vi "stepper driver -- IMS -- V2.vi"(7 "stepper driver action":T3, 8 "internal stepper driver state IMS":T1={"VISA address"="GPIB0::25::INSTR", "stepper motor state"=enum."stopped", "Motor Address"=0, "speed"=0, "target position"=0.0, "current position"=0.0}, 11 "number":dbl format="%#_13g") -> (0 "internal stepper driver state IMS -- OUT":T1={"VISA address"="GPIB0::25::INSTR", "stepper motor state"=enum."stopped", "Motor Address"=0, "speed"=0, "target position"=0.0, "current position"=0.0}, 1 "stepper motor state OUT":T2, 3 "current position":dbl)   [LabVIEW 2018]
uses:
  stepper motor action.ctl
  stepper motor state.ctl
  internal stepper driver state -- IMS.ctl
  stack action -- control.ctl
  Q - not nan -- integer.vi
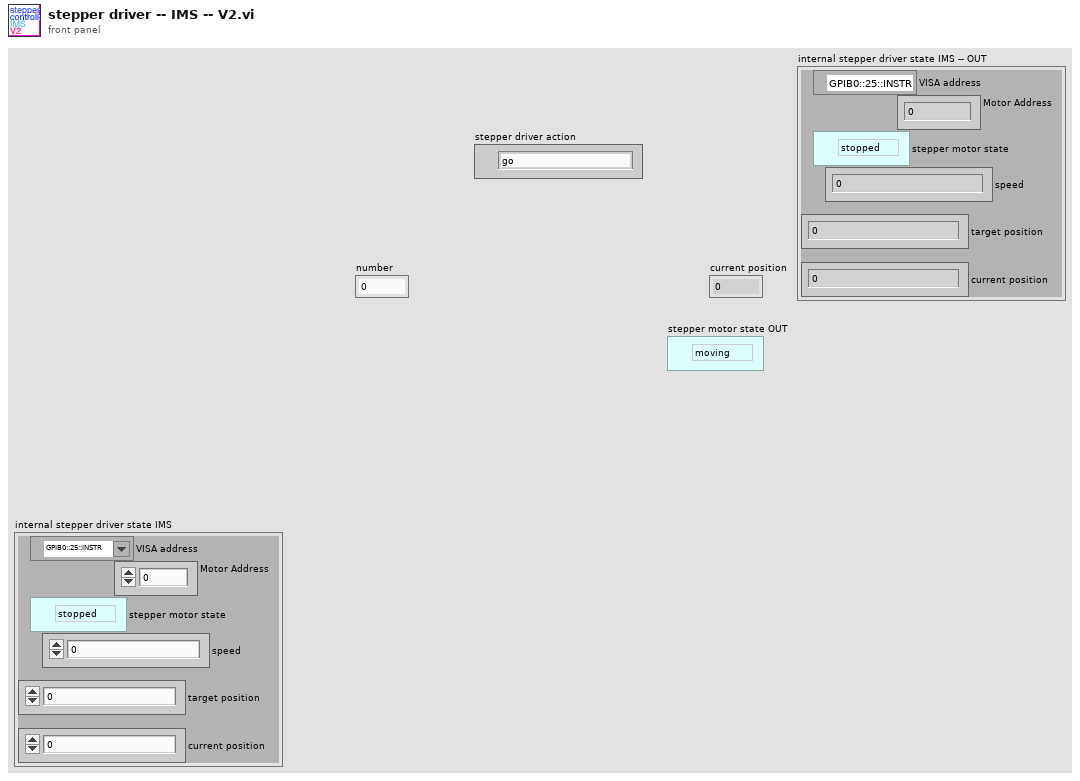
[diagram p1: front panel]
types:
  T1 = typedef "internal stepper driver state -- IMS.ctl" = cluster{"VISA address":refnum<visa-resource-name>, "stepper motor state":T2, "Motor Address":u32, "speed":i32, "target position":dbl, "current position":dbl}
  T2 = typedef "stepper motor state.ctl" = enum16{"moving", "stopped"}
  T3 = typedef "stepper motor action.ctl" = enum16{"go", "void", "stop", "check", "init", "sync", "set", "set speed", "--check status", "--check value"}
  T4 = typedef "stack action -- control.ctl" = enum16{"push", "pop", "check", "init"}
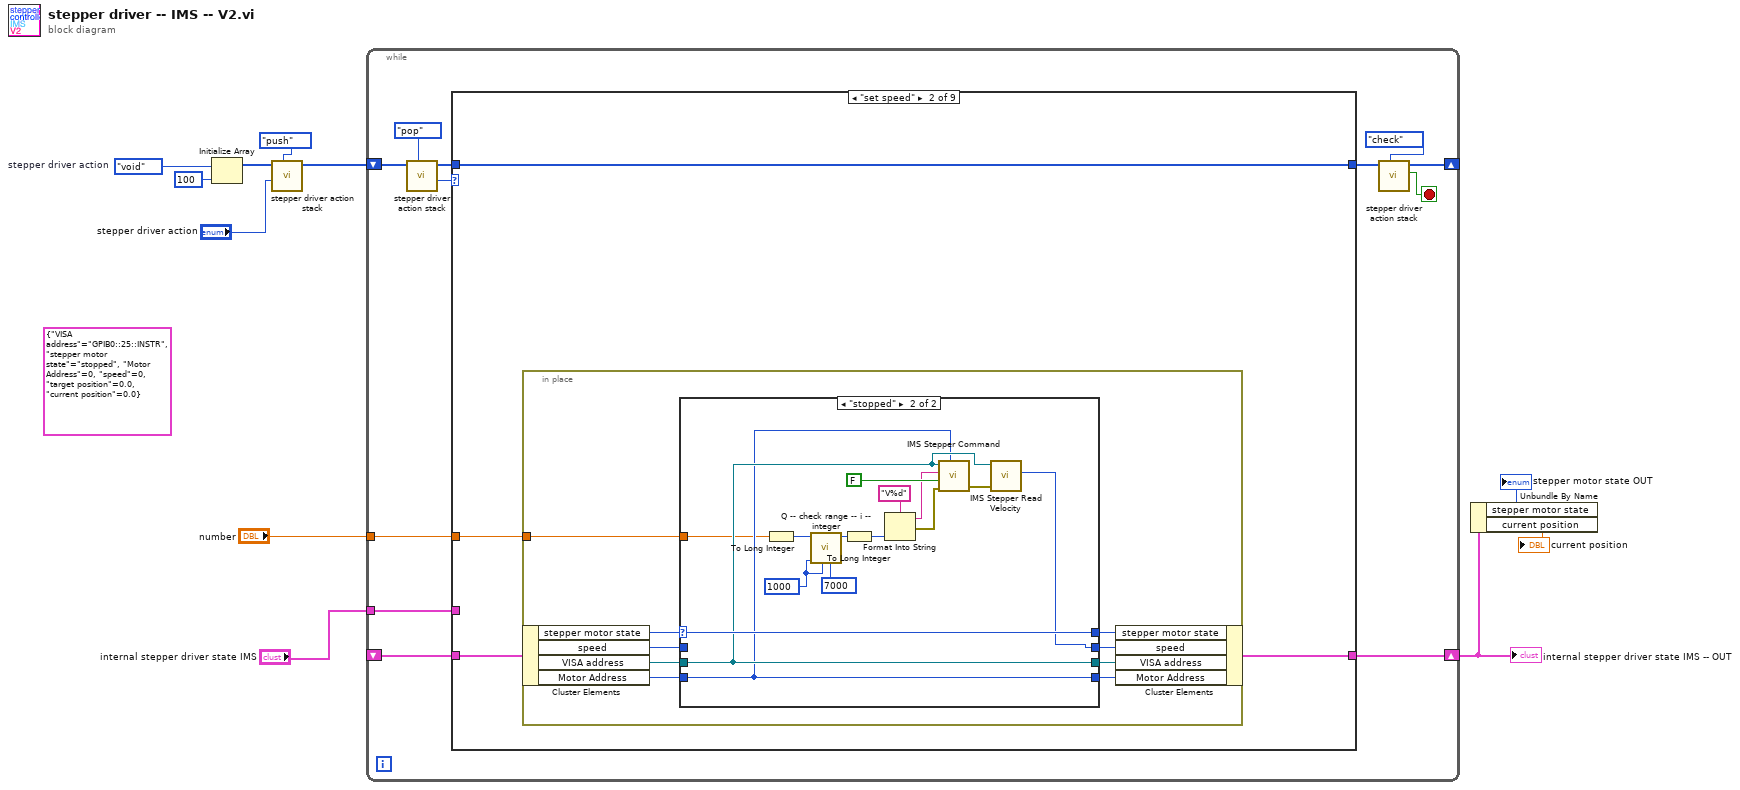
[diagram p0: block diagram]
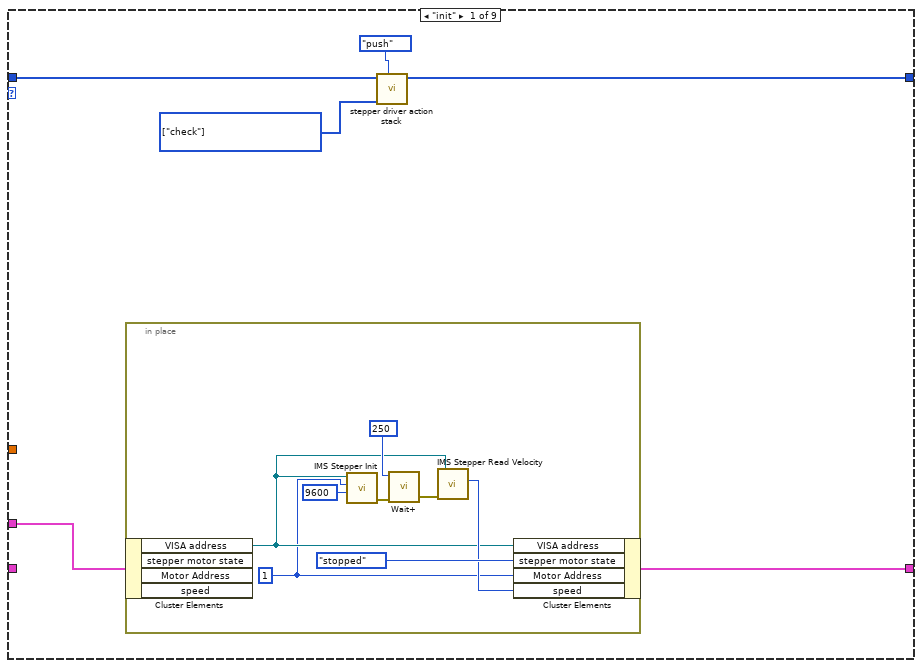
[diagram p2: hidden frame]
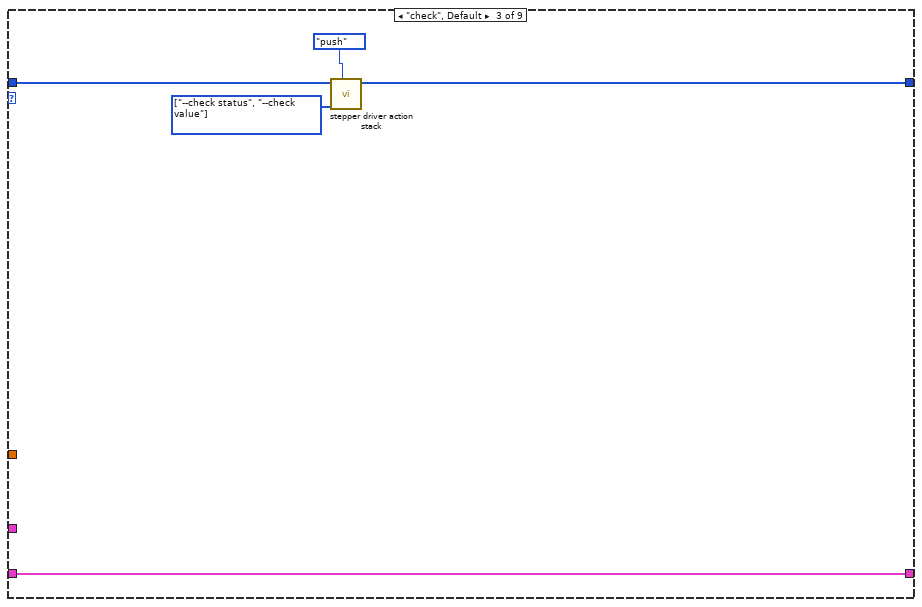
[diagram p4: hidden frame]
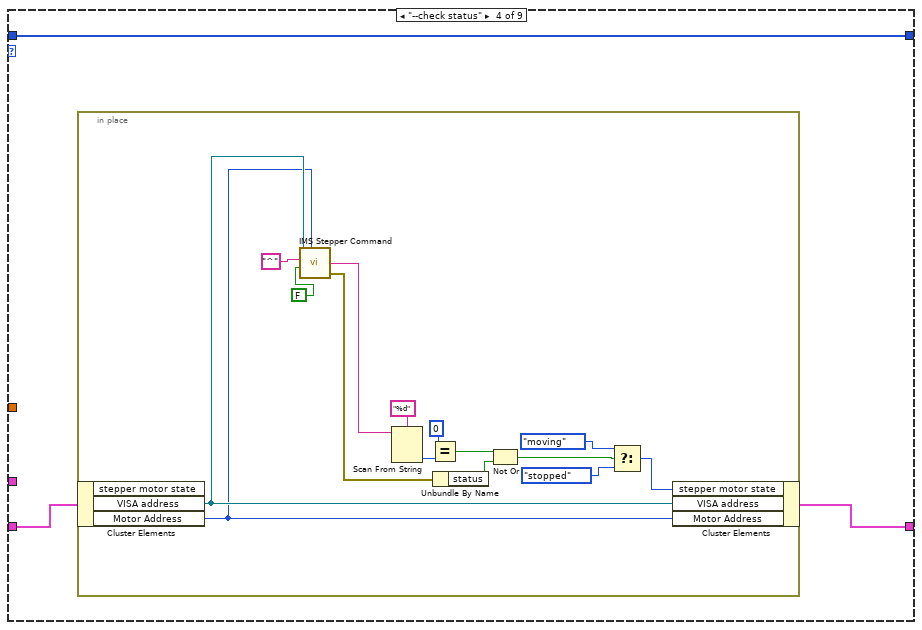
[diagram p5: hidden frame]
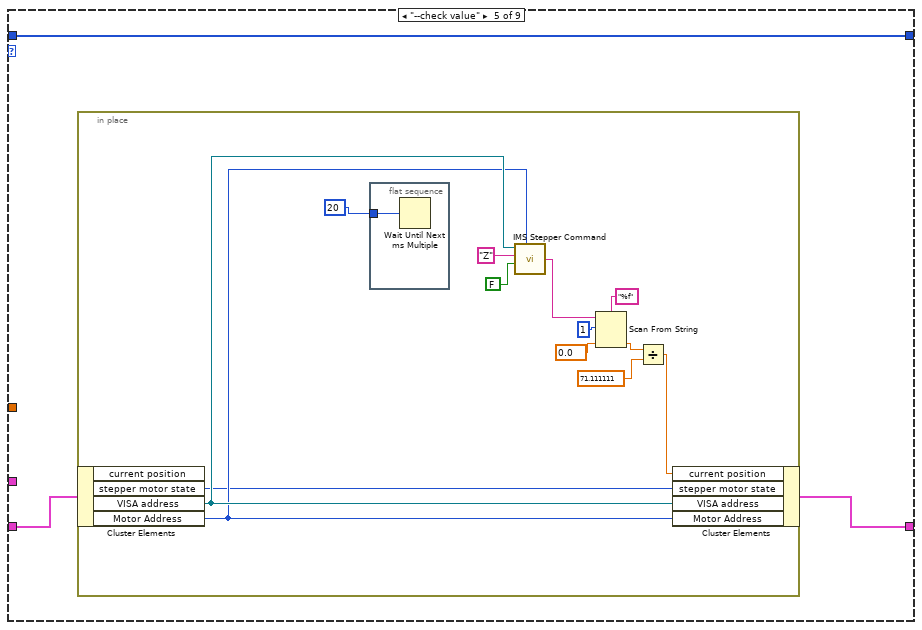
[diagram p6: hidden frame]
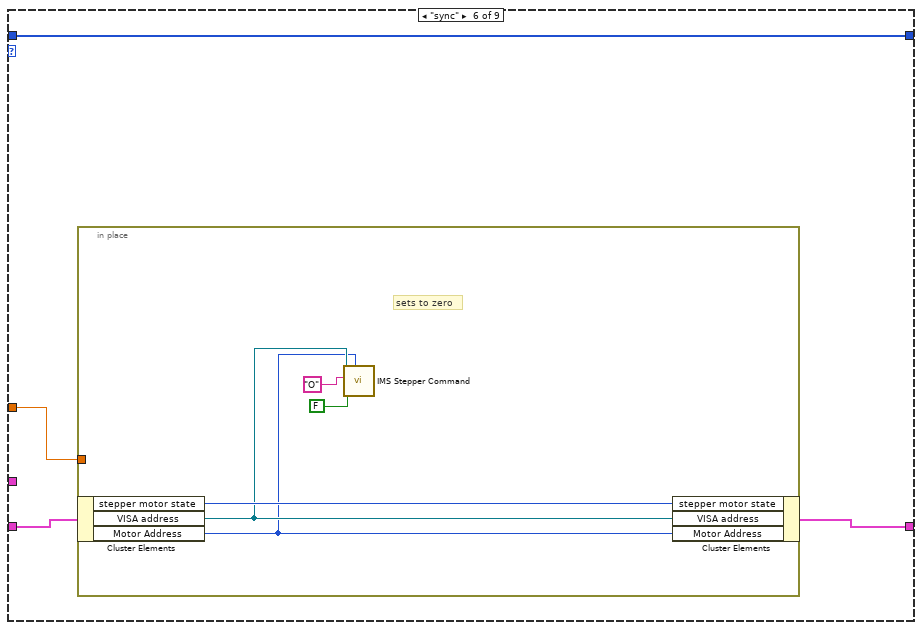
[diagram p7: hidden frame]
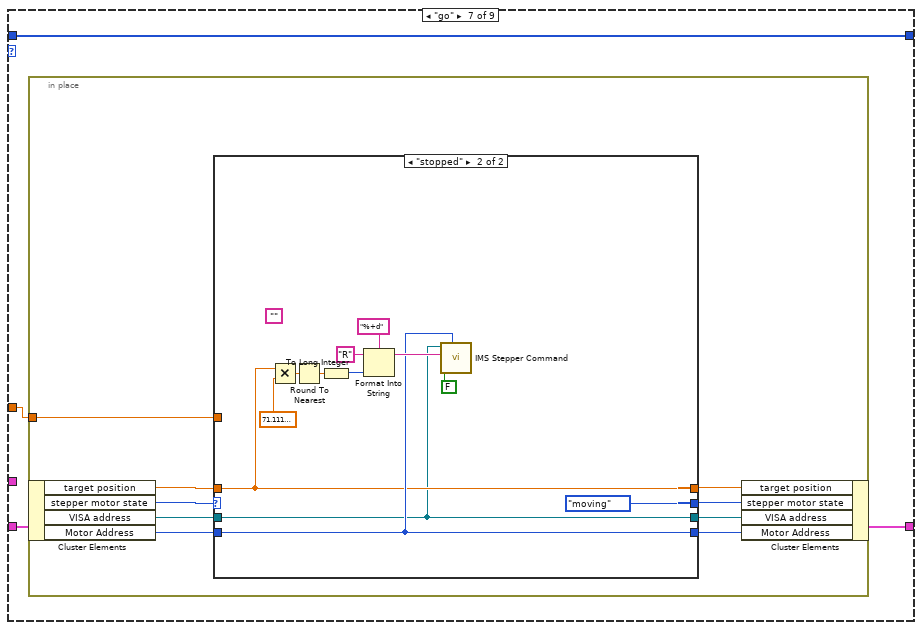
[diagram p8: hidden frame]
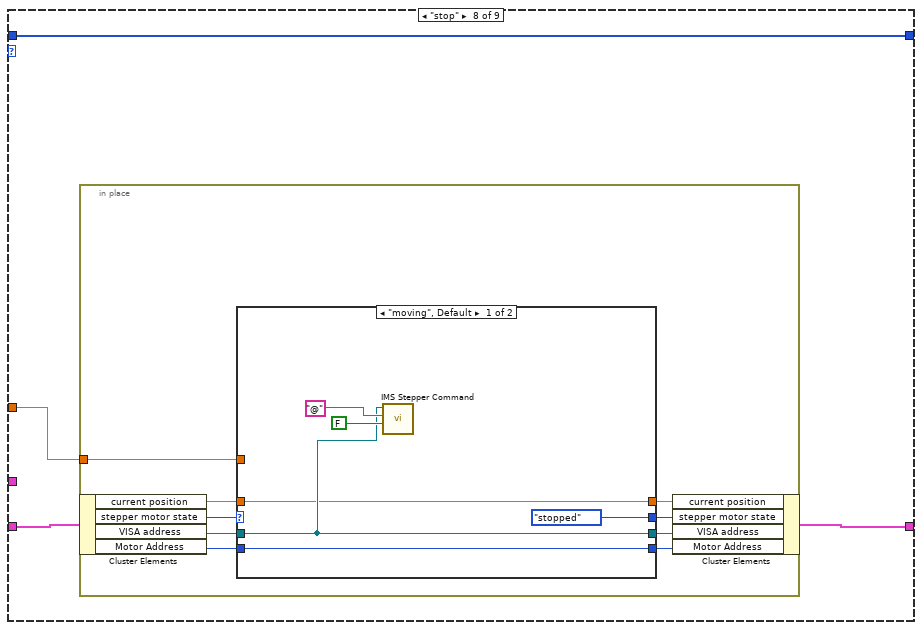
[diagram p10: hidden frame]
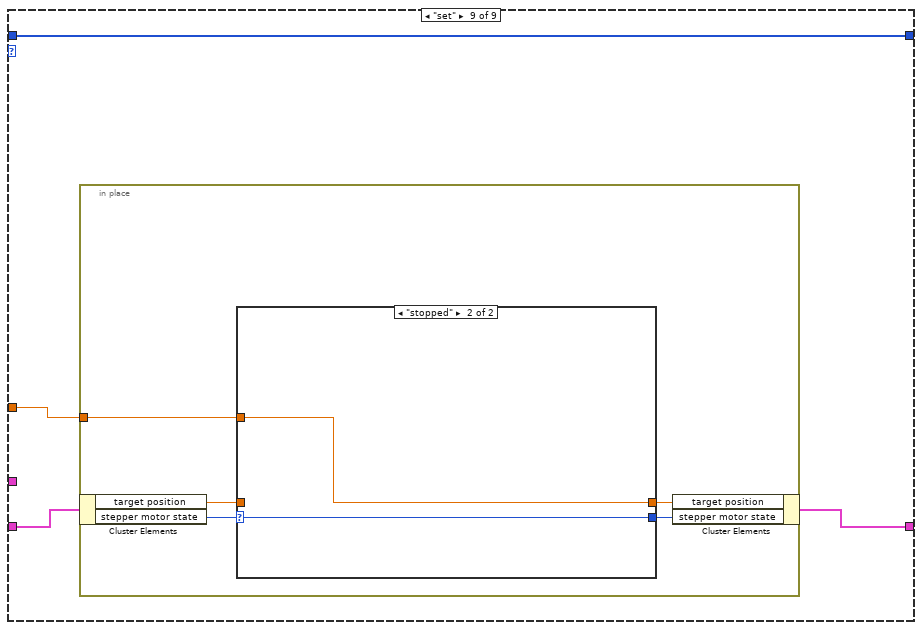
[diagram p12: hidden frame]
diagram:
  (unwired) T1 {"VISA address"="GPIB0::25::INSTR", "stepper motor state"=enum."stopped", "Motor Address"=0, "speed"=0, "target position"=0.0, "current position"=0.0} ("internal stepper driver state IMS")
  w11 = stepper_motor_action."void"  # stepper driver action
  n1 = Initialize Array(w11, 100 ("dimension size")) -> (w9:T3[])
  n2 = call "stepper driver action stack.vi"("stack action"=stack_action_--_control."push", "stepper driver action IN"="stepper driver action", "stack IN"=w9) -> ("command stack OUT"=w1:T3[])  [unwired: 6 in, 2 out]
  n3 = while {
    shift-right: [w23] -> w2
    shift-left: _ -> [w22]
    shift-right: [w16] -> _
    shift-left: w1 -> [w20]
    tunnel: "internal stepper driver state IMS" -> [w13]
    tunnel: "number" -> [w12]
    stop <- w14 stop-if-true
    n4 = call "stepper driver action stack.vi"("stack action"=stack_action_--_control."pop", "stack IN"=w20) -> ("stepper driver action  OUT"=w19:T3, "command stack OUT"=w18:T3[])  [unwired: 7 in, 1 out]
    n5 = case shown="\"set speed\"" w19 {
      tunnel: [w28 w39 w70 w76 w94 w111 w120 w149 w172] -> w23
      tunnel: w22 -> [_ w40 w70 w77 w95 w112 w121 w150 w173]
      tunnel: [w25 w41 w72 w75 w93 w113 w122 w151 w174] -> w17
      tunnel: w18 -> [w26 w41 w73 w75 w93 w113 w122 w151 w174]
      tunnel: w13 -> [w29 _ _ _ _ _ _ _ _]
      tunnel: w12 -> [_ w38 _ _ _ w110 w119 w148 w171]
      frame "init" {
        w24 = T3[] [enum."check"] items=["go", "void", "stop", "check", "init", "sync", "set", "set speed", "--check status", "--check value"] ("action list IN")
        n6 = in-place {
          w30 = u32 1 ("Motor Address")
          n7 = in-place-cluster #1(w29) -> ("VISA address"=w31:refnum<visa-resource-name>)  [unwired: 3 out]
          n8 = call "IMS Stepper Init.vi"("Baud Rate"=u32 9600, "Motor Number"=w30, "Instrument Address"=w31) -> ("error out"=w36:errorcluster)  [unwired: 1 in, 1 out]
          n9 = call "Wait+.vi"("Error In"=w36, "milliseconds to wait"=u32 250) -> ("Error Out"=w35:errorcluster)  [unwired: 4 in, 1 out]
          n10 = call "IMS Stepper Read Velocity.vi"("error in (no error)"=w35, "Instrument Address"=w31) -> ("Velocity"=w32:i32)  [unwired: 3 in, 2 out]
          n11 = in-place-cluster #1("VISA address"=w31, "stepper motor state"=stepper_motor_state."stopped", "Motor Address"=w30, "speed"=w32) -> (w28:T1)
        }
        n12 = call "stepper driver action stack.vi"("stack action"=stack_action_--_control."push", "action list IN"=w24, "stack IN"=w26) -> ("command stack OUT"=w25:T3[])  [unwired: 6 in, 2 out]
      }
      frame "set speed" {
        n13 = in-place {
          in-place-border: w38 -> [w50]
          n14 = in-place-cluster #2(w40) -> ("stepper motor state"=w46:T2, "speed"=w45:i32, "VISA address"=w48:refnum<visa-resource-name>, "Motor Address"=w47:u32)
          n15 = case shown="\"stopped\"" w46 {
            selector: w46 -> [w51 w67]
            tunnel: w50 -> [_ w56]
            tunnel: [w54 w58] -> w49
            tunnel: w48 -> [w53 w59]
            tunnel: w47 -> [w52 w57]
            tunnel: w45 -> [w54 _]
            tunnel: [w53 w59] -> w44
            tunnel: [w52 w57] -> w43
            tunnel: [w51 w67] -> w42
            frame "moving", Default {
            }
            frame "stopped" {
              w69 = 1000 ("lower limit")
              n16 = To Long Integer(number=w56) -> (32bit integer=w55:i32)
              n17 = call "Q -- check range -- i -- integer.vi"("upper"=7000 ("x"), "lower"=w69, "default"=w69, "number"=w55) -> ("number in range"=w61:i32)  [unwired: 5 in, 2 out]
              n18 = To Long Integer(number=w61) -> (32bit integer=w60:i32)
              n19 = Format Into String(format string="V%d", w60) -> (resulting string=w64:string, error out=w63:errorcluster)  [unwired: 2 in]
              n20 = call "IMS Stepper Command.vi"("Instrument Address"=w59, "Motor Number"=w57, "Command"=w64, "Mode"=FALSE, "error in (no error)"=w63) -> ("error out"=w62:errorcluster)  [unwired: 1 in, 2 out]
              n21 = call "IMS Stepper Read Velocity.vi"("error in (no error)"=w62, "Instrument Address"=w59) -> ("Velocity"=w58:i32)  [unwired: 3 in, 2 out]
            }
          }
          n22 = in-place-cluster #2("stepper motor state"=w42, "speed"=w49, "VISA address"=w44, "Motor Address"=w43) -> (w39:T1)
        }
      }
      frame "check", Default {
        w71 = T3[] [enum."--check status", enum."--check value"] items=["go", "void", "stop", "check", "init", "sync", "set", "set speed", "--check status", "--check value"] ("action list IN")
        n23 = call "stepper driver action stack.vi"("stack action"=stack_action_--_control."push", "action list IN"=w71, "stack IN"=w73) -> ("command stack OUT"=w72:T3[])  [unwired: 6 in, 2 out]
      }
      frame "--check status" {
        n24 = in-place {
          n25 = in-place-cluster #3(w77) -> ("VISA address"=w80:refnum<visa-resource-name>, "Motor Address"=w79:u32)  [unwired: 1 out]
          n26 = call "IMS Stepper Command.vi"("Instrument Address"=w80, "Motor Number"=w79, "Command"="^", "Mode"=FALSE) -> ("Response"=w87:string, "error out"=w78:errorcluster)  [unwired: 2 in, 1 out]
          n27 = Scan From String(format string="%d", input string=w87) -> (output 1=w88:i32)  [unwired: 3 in, 3 out]
          n28 = Equal?(x=0, y=w88) -> (x = y?=w89:bool)
          n29 = Unbundle By Name(w78) -> ("status"=w90:bool)
          n30 = Not Or(1:w90, 2:w89) -> (0:w82:bool)
          n31 = Select(t=stepper_motor_state."moving" ("stepper motor state"), s=w82, f=stepper_motor_state."stopped" ("stepper motor state")) -> (s? t:f=w81:T2)
          n32 = in-place-cluster #3("stepper motor state"=w81, "VISA address"=w80, "Motor Address"=w79) -> (w76:T1)
        }
      }
      frame "--check value" {
        n33 = in-place {
          n34 = in-place-cluster #4(w95) -> ("stepper motor state"=w96:T2, "VISA address"=w100:refnum<visa-resource-name>, "Motor Address"=w99:u32)  [unwired: 1 out]
          n35 = flat-sequence {
            tunnel: u32 20 ("millisecond multiple") -> [w109]
            frame #0 {
              n36 = Wait Until Next ms Multiple(millisecond multiple=w109) -> ()  [unwired: 1 out]
            }
          }
          n37 = call "IMS Stepper Command.vi"("Instrument Address"=w100, "Motor Number"=w99, "Command"="Z", "Mode"=FALSE) -> ("Response"=w105:string)  [unwired: 2 in, 2 out]
          n38 = Scan From String(format string="%f", input string=w105, initial scan location=u32 1, default 1=0.0 ("default value 1")) -> (output 1=w107:dbl)  [unwired: 1 in, 3 out]
          n39 = Divide(x=w107, y=71.111111) -> (x/y=w98:dbl)
          n40 = in-place-cluster #4("current position"=w98, "stepper motor state"=w96, "VISA address"=w100, "Motor Address"=w99) -> (w94:T1)
        }
      }
      frame "sync" {
        n41 = in-place {
          in-place-border: w110 -> [_]
          # "sets to zero"
          n42 = in-place-cluster #5(w112) -> ("stepper motor state"=w118:T2, "VISA address"=w115:refnum<visa-resource-name>, "Motor Address"=w114:u32)
          n43 = call "IMS Stepper Command.vi"("Instrument Address"=w115, "Motor Number"=w114, "Command"="O", "Mode"=FALSE) -> ()  [unwired: 2 in, 3 out]
          n44 = in-place-cluster #5("stepper motor state"=w118, "VISA address"=w115, "Motor Address"=w114) -> (w111:T1)
        }
      }
      frame "go" {
        n45 = in-place {
          in-place-border: w119 -> [w131]
          n46 = in-place-cluster #6(w121) -> ("target position"=w125:dbl, "stepper motor state"=w128:T2, "VISA address"=w130:refnum<visa-resource-name>, "Motor Address"=w129:u32)
          n47 = case shown="\"stopped\"" w128 {
            selector: w128 -> [w132 _]
            tunnel: w131 -> [_ _]
            tunnel: w130 -> [w135 w137]
            tunnel: w129 -> [w134 w139]
            tunnel: [w135 w137] -> w127
            tunnel: [w134 w139] -> w126
            tunnel: w125 -> [w133 w138]
            tunnel: [w132 stepper_motor_state."moving" ("stepper motor state")] -> w124
            tunnel: [w133 w138] -> w123
            frame "moving", Default {
            }
            frame "stopped" {
              (unwired) ""
              n48 = Multiply(x=w138, y=71.11111111) -> (x*y=w145:dbl)
              n49 = Round To Nearest(number=w145) -> (nearest integer value=w143:dbl)
              n50 = To Long Integer(number=w143) -> (32bit integer=w144:i32)
              n51 = Format Into String(format string="%+d", initial string="R", w144) -> (resulting string=w140:string)  [unwired: 1 in, 1 out]
              n52 = call "IMS Stepper Command.vi"("Instrument Address"=w137, "Motor Number"=w139, "Command"=w140, "Mode"=FALSE) -> ()  [unwired: 2 in, 3 out]
            }
          }
          n53 = in-place-cluster #6("target position"=w123, "stepper motor state"=w124, "VISA address"=w127, "Motor Address"=w126) -> (w120:T1)
        }
      }
      frame "stop" {
        n54 = in-place {
          in-place-border: w148 -> [w160]
          n55 = in-place-cluster #7(w150) -> ("current position"=w152:dbl, "stepper motor state"=w157:T2, "VISA address"=w159:refnum<visa-resource-name>, "Motor Address"=w158:u32)
          n56 = case shown="\"moving\", Default" w157 {
            selector: w157 -> [_ w168]
            tunnel: w160 -> [_ _]
            tunnel: w159 -> [w162 w170]
            tunnel: w158 -> [w166 w169]
            tunnel: [w162 w170] -> w156
            tunnel: [w166 w169] -> w155
            tunnel: [stepper_motor_state."stopped" ("stepper motor state") w168] -> w154
            tunnel: [w161 w167] -> w153
            tunnel: w152 -> [w161 w167]
            frame "moving", Default {
              n57 = call "IMS Stepper Command.vi"("Instrument Address"=w162, "Command"="@", "Mode"=FALSE) -> ()  [unwired: 3 in, 3 out]
            }
            frame "stopped" {
            }
          }
          n58 = in-place-cluster #7("current position"=w153, "stepper motor state"=w154, "VISA address"=w156, "Motor Address"=w155) -> (w149:T1)
        }
      }
      frame "set" {
        n59 = in-place {
          in-place-border: w171 -> [w179]
          n60 = in-place-cluster #8(w173) -> ("target position"=w175:dbl, "stepper motor state"=w178:T2)
          n61 = case shown="\"stopped\"" w178 {
            selector: w178 -> [w181 w183]
            tunnel: w179 -> [_ w182]
            tunnel: [w181 w183] -> w177
            tunnel: [w180 w182] -> w176
            tunnel: w175 -> [w180 _]
            frame "moving", Default {
            }
            frame "stopped" {
            }
          }
          n62 = in-place-cluster #8("target position"=w176, "stepper motor state"=w177) -> (w172:T1)
        }
      }
    }
    n63 = call "stepper driver action stack.vi"("stack action"=stack_action_--_control."check", "stack IN"=w17) -> ("stack is empty ?"=w14:bool, "command stack OUT"=w16:T3[])  [unwired: 7 in, 1 out]
  }
  "internal stepper driver state IMS -- OUT" <- w2
  n64 = Unbundle By Name(w2) -> ("stepper motor state"=→"stepper motor state OUT":T2, "current position"=→"current position":dbl)
